vi "main.vi"() -> ()   [LabVIEW 2023, in "Lavatory_Management.lvlib"]
doc: "Airplane lavatory simulator"
uses:
  Lavatory_Management.lvlib
  Controls/Queue Opertaions.ctl
  Controls/Managemet_data.ctl
  Controls/Lavatory_data.ctl
  Queue_Driver.lvlib
panel:
  out "Alarm Time D":dbl caption="Secs" format="%#.3g"
  out "Alarm Time C":dbl caption="Secs" format="%#.3g"
  out "Alarm Time B":dbl caption="Secs" format="%#.3g"
  out "Alarm Time A":dbl caption="Secs" format="%#.3g"
  in  "error in (no error)":errorcluster
  in  "Stop simulation":bool
  in  "Alarm Timer Limit":i32=10 caption="secs" min=1 max=120 step=1
  in  "Lavatory D Occupied":bool
  in  "Lavatory B Occupied":bool
  in  "Lavatory C Occupied":bool
  in  "Lavatory A Occupied":bool
  in  "Alarm Acknowledge":bool
  out "Lavatory":string
  out "Alarm":bool
  in  "Seatbelt Sign ON":bool
  out "Lavatories_Occupied_Rear":bool caption="Lavatories \nOccupied"
  out "Lavatories_Occupied_Front":bool caption="Lavatories \nOccupied"
  out "Return_to_seat_d":bool caption="Return to seat"
  out "Return_to_seat_b":bool caption="Return to seat"
  out "Return_to_seat_c":bool caption="Return to seat"
  out "Return_to_seat_a":bool caption="Return to seat"
  out "Occupied_C":bool caption="Occupied C"
  out "Occupied_D":bool caption="Occupied D"
  out "Occupied_B":bool caption="Occupied B"
  out "Occupied_A":bool caption="Occupied A"
  # "Airplane Lavatory Signs"
  # "Front"
  # "Rear"
  # "Lavatory A"
  # "Lavatory C"
  # "Lavatory B"
  # "Lavatory D"
  # "Simulation Controls & Indicators"
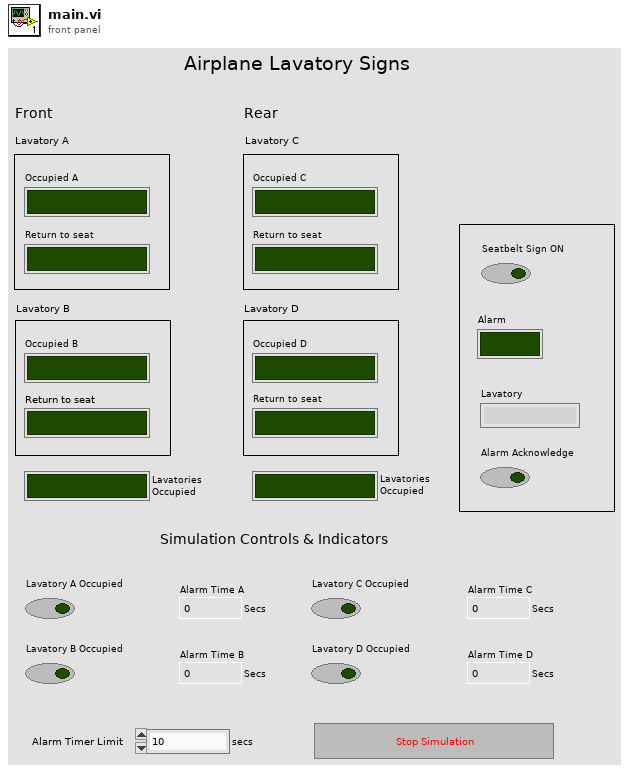
[diagram p1: front panel]
types:
  T1 = typedef "Lavatory_Management.lvlib/Managemet_data.ctl" = cluster{"Lavatory_A":T2, "Lavatory_B":T2, "Lavatory_C":T2, "Lavatory_D":T2, "Seat_belt":bool, "Alarm":bool, "Lavatory":string, "Timr_Limit":i32, "Time_Now":timestamp}
  T2 = typedef "Lavatory_Management.lvlib/Lavatory_data.ctl" = cluster{"Timer":timestamp, "Occupied":bool}
  T3 = typedef "Queue_Driver.lvlib/Queue Opertaions.ctl" = enum16{"Create", "Enqueue", "Enqueue N", "Flush", "Dequeue", "Destroy"}
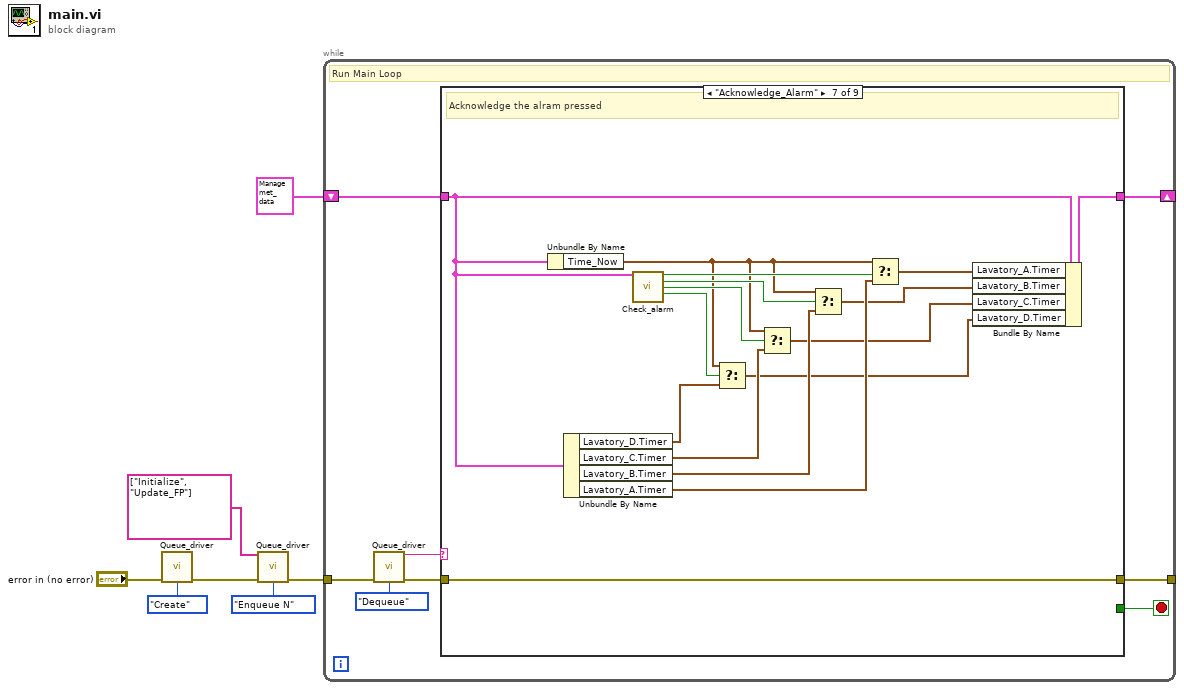
[diagram p0: block diagram]
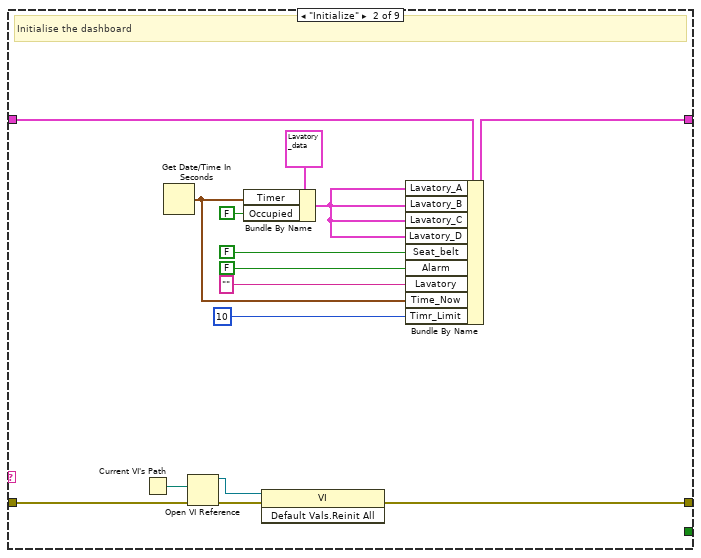
[diagram p3: hidden frame]
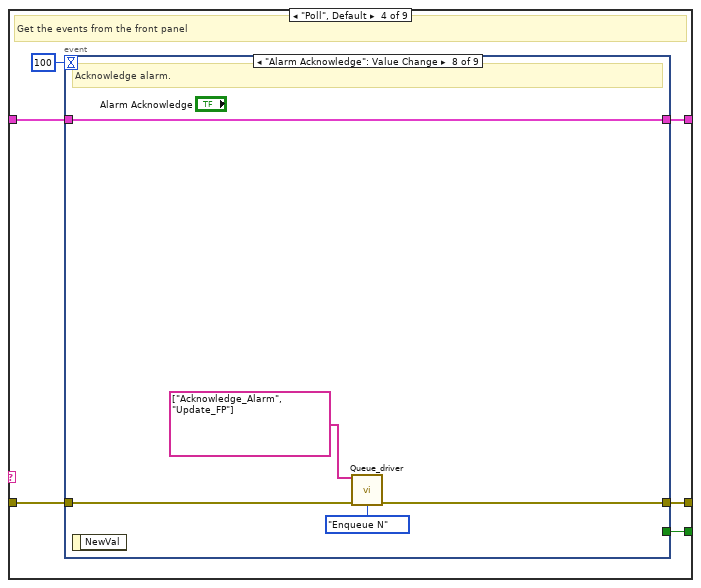
[diagram p5: hidden frame]
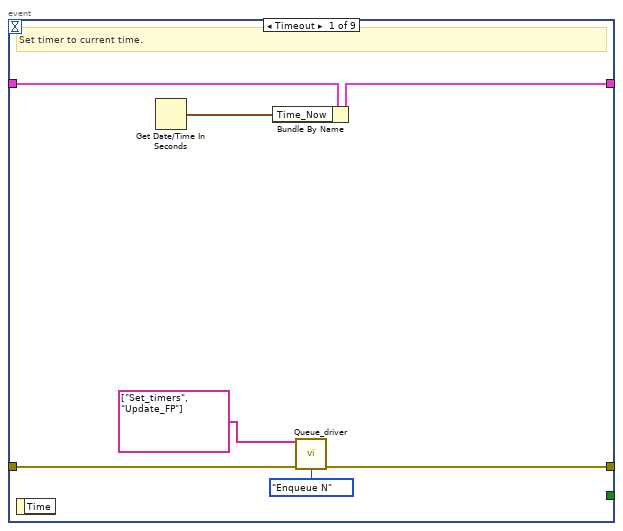
[diagram p6: hidden frame]
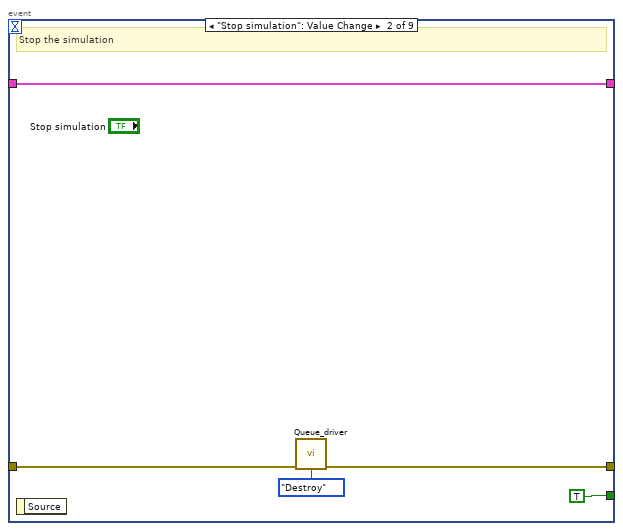
[diagram p7: hidden frame]
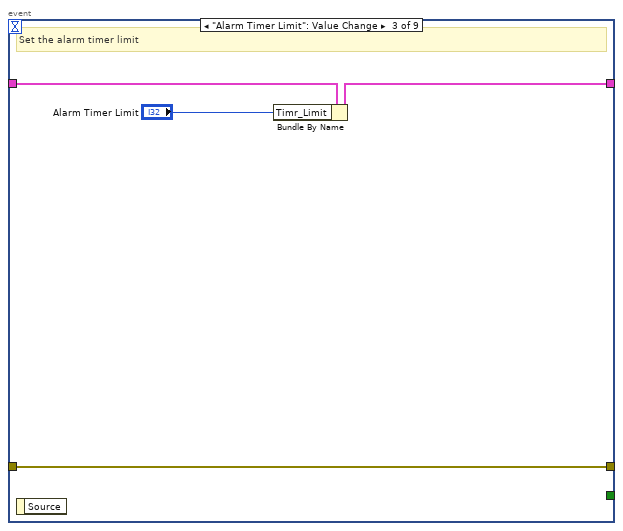
[diagram p8: hidden frame]
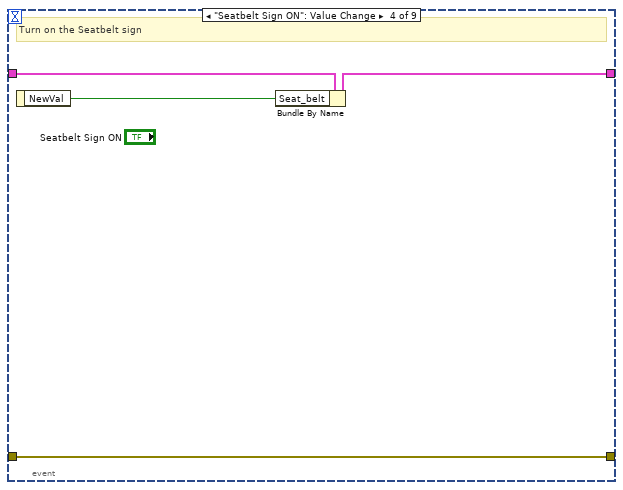
[diagram p9: hidden frame]
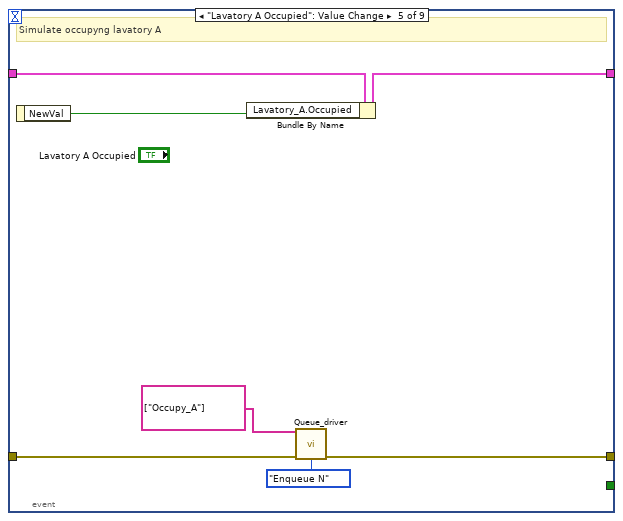
[diagram p10: hidden frame]
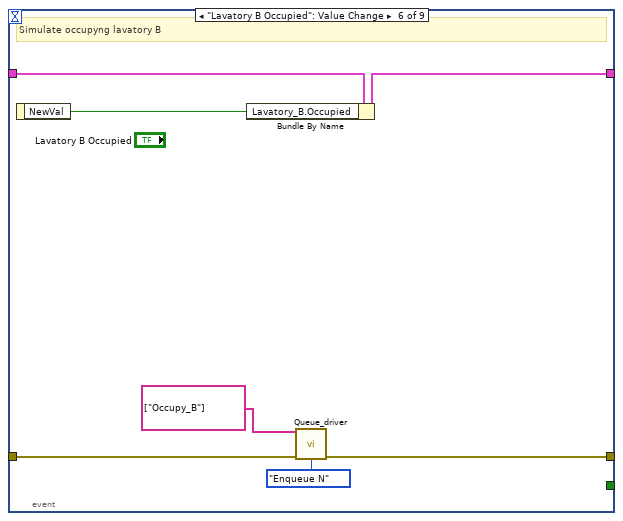
[diagram p11: hidden frame]
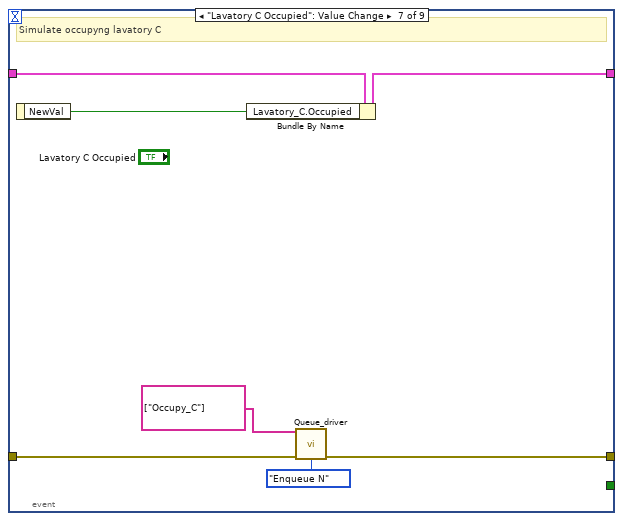
[diagram p12: hidden frame]
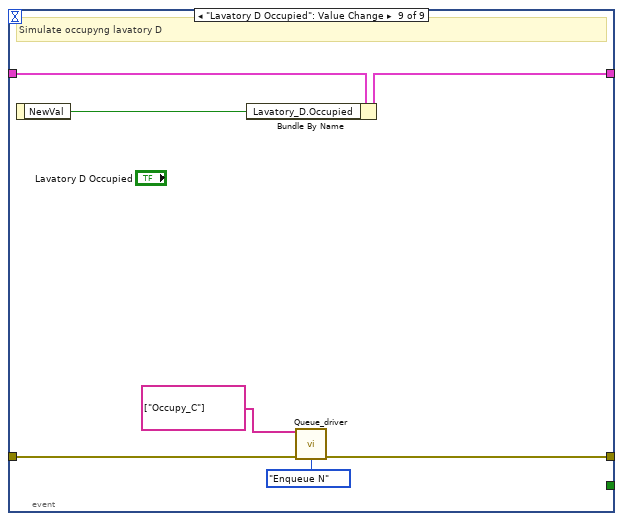
[diagram p13: hidden frame]
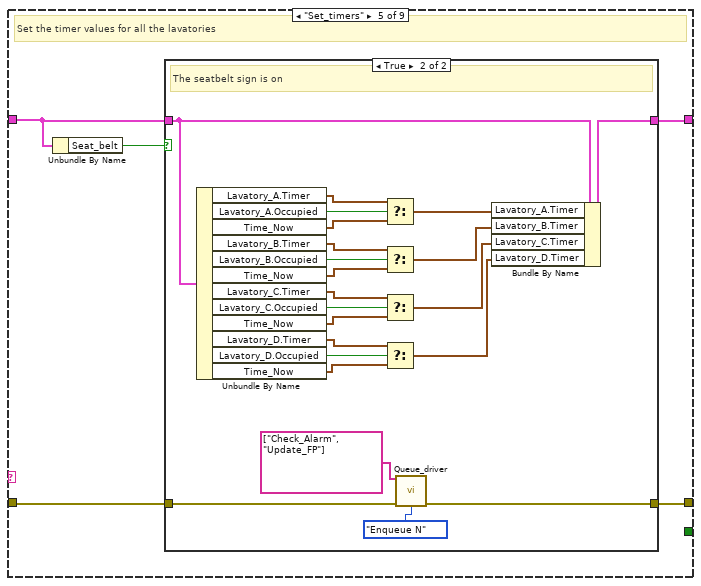
[diagram p14: hidden frame]
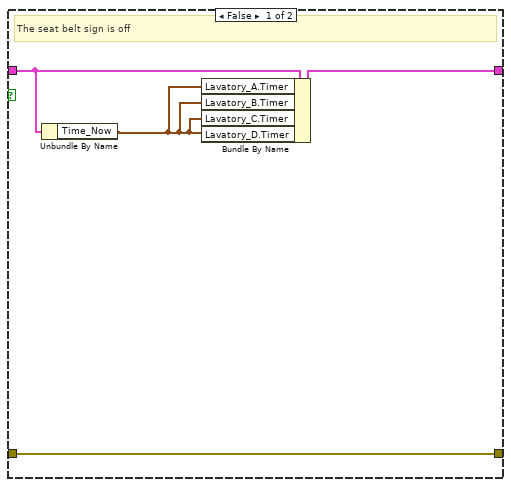
[diagram p15: hidden frame]
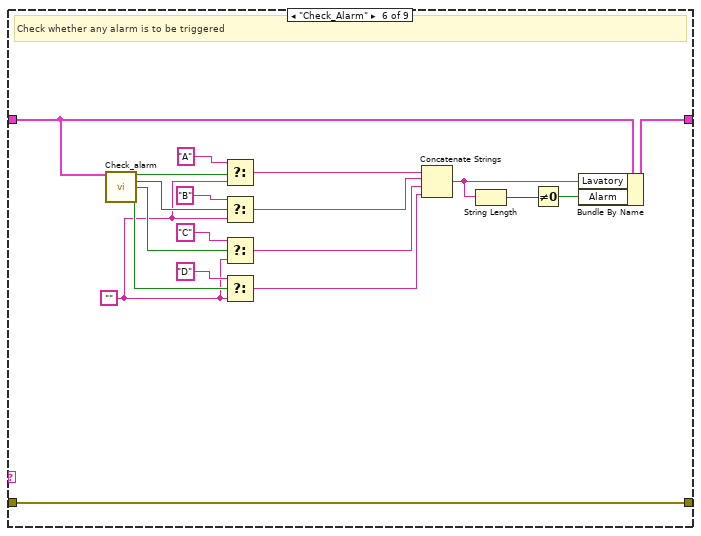
[diagram p16: hidden frame]
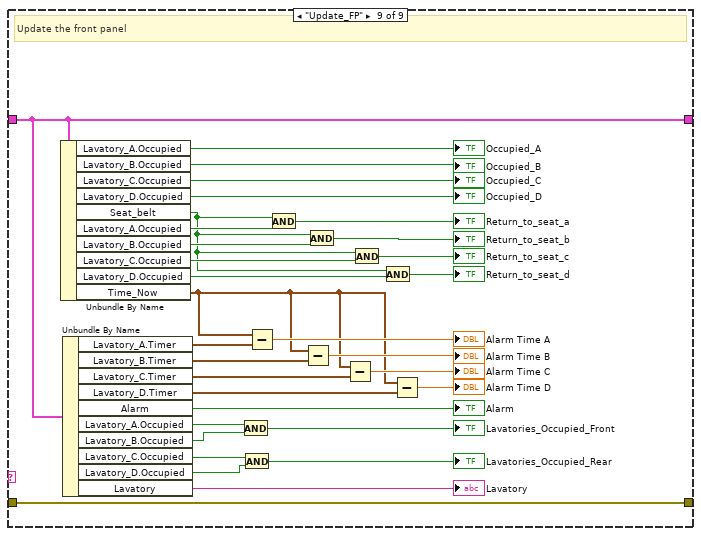
[diagram p18: hidden frame]
diagram:
  n1 = call "Queue_driver.vi"("error in (no error)"="error in (no error)", "Operations"=Queue_Opertaions."Create") -> ("error out"=w5:errorcluster)  [unwired: 12 in, 1 out]
  n2 = call "Queue_driver.vi"("Array Elements"=string[] ["Initialize", "Update_FP"], "error in (no error)"=w5, "Operations"=Queue_Opertaions."Enqueue N") -> ("error out"=w4:errorcluster)  [unwired: 11 in, 1 out]
  n3 = while {
    tunnel: w4 -> [w15]
    tunnel: [w12] -> _
    shift-right: [w9] -> _
    shift-left: T1 {"Lavatory_A"={"Timer"=timestamp(0 s since 1904-01-01), "Occupied"=FALSE}, "Lavatory_B"={"Timer"=timestamp(0 s since 1904-01-01), "Occupied"=FALSE}, "Lavatory_C"={"Timer"=timestamp(0 s since 1904-01-01), "Occupied"=FALSE}, "Lavatory_D"={"Timer"=timestamp(0 s since 1904-01-01), "Occupied"=FALSE}, "Seat_belt"=TRUE, "Alarm"=TRUE, "Lavatory"="", "Timr_Limit"=0, "Time_Now"=timestamp(0 s since 1904-01-01)} -> [w10]
    stop <- w8 stop-if-true
    # "Run Main Loop"
    n4 = call "Queue_driver.vi"("error in (no error)"=w15, "Operations"=Queue_Opertaions."Dequeue") -> ("Element out"=w11:string, "error out"=w13:errorcluster)  [unwired: 12 in]
    n5 = case shown="\"Acknowledge_Alarm\"" w11 {
      tunnel: [w16 w22 w33 w40 w95 w143 w144 w160 w165] -> w12
      tunnel: w13 -> [w16 w32 w33 w39 w94 w143 w144 w160 w165]
      tunnel: w10 -> [w17 w31 w34 w38 w96 w142 w158 w161 w178]
      tunnel: [w17 w30 w34 w37 w97 w141 w149 w161 w178] -> w9
      tunnel: [_ _ _ w36 _ _ _ _ _] -> w8
      frame "/***init***/" {
        # "Contains initialising states"
      }
      frame "Initialize" {
        # "Initialise the dashboard"
        n6 = Current VI's Path() -> (path=w23:path)
        n7 = Get Date/Time In Seconds() -> (seconds since 1Jan1904=w19:timestamp)
        n8 = Open VI Reference(vi path=w23, error in (no error)=w32) -> (vi reference=w21:refnum<vi>, error out=w24:errorcluster)  [unwired: 4 in]
        n9 = Bundle By Name(cluster=T2 {"Timer"=timestamp(0 s since 1904-01-01), "Occupied"=FALSE} ("Cluster"), "Timer"=w19, "Occupied"=FALSE) -> (w25:T2)
        n10 = invoke class="VI" method="Default Vals.Reinit All"(reference=w21, error in=w24) -> (error out=w22:errorcluster)  [unwired: 1 in, 2 out]
        n11 = Bundle By Name(cluster=w31, "Lavatory_A"=w25, "Lavatory_B"=w25, "Lavatory_C"=w25, "Lavatory_D"=w25, "Seat_belt"=FALSE, "Alarm"=FALSE, "Lavatory"="", "Time_Now"=w19, "Timr_Limit"=10) -> (w30:T1)
      }
      frame "/***Functionality***/" {
      }
      frame "Poll", Default {
        # "Get the events from the front panel"
        n12 = event shown="[7] \"Alarm Acknowledge\": Value Change" {
          selector: _ -> [_ _ _ _ _ _ _ _ _]
          dyn-events: _ -> [_ _ _ _ _ _ _ _ _]
          timeout: 100 -> [_ _ _ _ _ _ _ _ _]
          tunnel: [w45 w49 w53 w59 w63 w70 w77 w84 w89] -> w40
          tunnel: w39 -> [w47 w51 w53 w59 w67 w74 w81 w85 w93]
          tunnel: w38 -> [w46 w50 w56 w60 w66 w73 w80 w86 w92]
          tunnel: [w42 w50 w55 w58 w65 w72 w79 w86 w91] -> w37
          tunnel: [_ TRUE _ _ _ _ _ _ _] -> w36
          event Timeout {
            # "Set timer to current time."
            n13 = event-data() -> ()  [unwired: 1 in, 1 out]
            n14 = Get Date/Time In Seconds() -> (seconds since 1Jan1904=w41:timestamp)
            n15 = Bundle By Name(cluster=w46, "Time_Now"=w41) -> (w42:T1)
            n16 = call "Queue_driver.vi"("Array Elements"=string[] ["Set_timers", "Update_FP"], "error in (no error)"=w47, "Operations"=Queue_Opertaions."Enqueue N") -> ("error out"=w45:errorcluster)  [unwired: 11 in, 1 out]
          }
          event "Stop simulation": Value Change {
            # "Stop the simulation"
            n17 = event-data() -> ()  [unwired: 1 in, 1 out]
            n18 = call "Queue_driver.vi"("error in (no error)"=w51, "Operations"=Queue_Opertaions."Destroy") -> ("error out"=w49:errorcluster)  [unwired: 12 in, 1 out]
          }
          event "Alarm Timer Limit": Value Change {
            # "Set the alarm timer limit"
            n19 = event-data() -> ()  [unwired: 1 in, 1 out]
            n20 = Bundle By Name(cluster=w56, "Timr_Limit"="Alarm Timer Limit") -> (w55:T1)
          }
          event "Seatbelt Sign ON": Value Change {
            # "Turn on the Seatbelt sign"
            n21 = event-data() -> ("NewVal"=w57:bool)  [unwired: 1 in]
            n22 = Bundle By Name(cluster=w60, "Seat_belt"=w57) -> (w58:T1)
          }
          event "Lavatory A Occupied": Value Change {
            # "Simulate occupyng lavatory A"
            n23 = event-data() -> ("NewVal"=w64:bool)  [unwired: 1 in]
            n24 = Bundle By Name(cluster=w66, "Lavatory_A.Occupied"=w64) -> (w65:T1)
            n25 = call "Queue_driver.vi"("Array Elements"=string[] ["Occupy_A"], "error in (no error)"=w67, "Operations"=Queue_Opertaions."Enqueue N") -> ("error out"=w63:errorcluster)  [unwired: 11 in, 1 out]
          }
          event "Lavatory B Occupied": Value Change {
            # "Simulate occupyng lavatory B"
            n26 = event-data() -> ("NewVal"=w71:bool)  [unwired: 1 in]
            n27 = Bundle By Name(cluster=w73, "Lavatory_B.Occupied"=w71) -> (w72:T1)
            n28 = call "Queue_driver.vi"("Array Elements"=string[] ["Occupy_B"], "error in (no error)"=w74, "Operations"=Queue_Opertaions."Enqueue N") -> ("error out"=w70:errorcluster)  [unwired: 11 in, 1 out]
          }
          event "Lavatory C Occupied": Value Change {
            # "Simulate occupyng lavatory C"
            n29 = event-data() -> ("NewVal"=w78:bool)  [unwired: 1 in]
            n30 = Bundle By Name(cluster=w80, "Lavatory_C.Occupied"=w78) -> (w79:T1)
            n31 = call "Queue_driver.vi"("Array Elements"=string[] ["Occupy_C"], "error in (no error)"=w81, "Operations"=Queue_Opertaions."Enqueue N") -> ("error out"=w77:errorcluster)  [unwired: 11 in, 1 out]
          }
          event "Alarm Acknowledge": Value Change {
            # "Acknowledge alarm."
            n32 = event-data() -> ()  [unwired: 1 in, 1 out]
            n33 = call "Queue_driver.vi"("Array Elements"=string[] ["Acknowledge_Alarm", "Update_FP"], "error in (no error)"=w85, "Operations"=Queue_Opertaions."Enqueue N") -> ("error out"=w84:errorcluster)  [unwired: 11 in, 1 out]
          }
          event "Lavatory D Occupied": Value Change {
            # "Simulate occupyng lavatory D"
            n34 = event-data() -> ("NewVal"=w90:bool)  [unwired: 1 in]
            n35 = Bundle By Name(cluster=w92, "Lavatory_D.Occupied"=w90) -> (w91:T1)
            n36 = call "Queue_driver.vi"("Array Elements"=string[] ["Occupy_C"], "error in (no error)"=w93, "Operations"=Queue_Opertaions."Enqueue N") -> ("error out"=w89:errorcluster)  [unwired: 11 in, 1 out]
          }
        }
      }
      frame "Set_timers" {
        # "Set the timer values for all the lavatories"
        n37 = Unbundle By Name(w96) -> ("Seat_belt"=w98:bool)
        n38 = case shown="True" w98 {
          tunnel: [w102 w121] -> w97
          tunnel: w96 -> [w100 w124]
          tunnel: [w101 w118] -> w95
          tunnel: w94 -> [w101 w119]
          frame False {
            # "The seat belt sign is off"
            n39 = Unbundle By Name(w100) -> ("Time_Now"=w99:timestamp)
            n40 = Bundle By Name(cluster=w100, "Lavatory_A.Timer"=w99, "Lavatory_B.Timer"=w99, "Lavatory_C.Timer"=w99, "Lavatory_D.Timer"=w99) -> (w102:T1)
          }
          frame True {
            # "The seatbelt sign is on"
            n41 = Unbundle By Name(w124) -> ("Lavatory_A.Timer"=w122:timestamp, "Lavatory_A.Occupied"=w123:bool, "Time_Now"=w116:timestamp, "Lavatory_B.Timer"=w115:timestamp, "Lavatory_B.Occupied"=w114:bool, "Time_Now"=w113:timestamp, "Lavatory_C.Timer"=w112:timestamp, "Lavatory_C.Occupied"=w111:bool, "Time_Now"=w110:timestamp, "Lavatory_D.Timer"=w109:timestamp, "Lavatory_D.Occupied"=w108:bool, "Time_Now"=w107:timestamp)
            n42 = Select(t=w122, s=w123, f=w116) -> (s? t:f=w120:timestamp)
            n43 = Select(t=w115, s=w114, f=w113) -> (s? t:f=w106:timestamp)
            n44 = Select(t=w112, s=w111, f=w110) -> (s? t:f=w105:timestamp)
            n45 = Select(t=w109, s=w108, f=w107) -> (s? t:f=w104:timestamp)
            n46 = call "Queue_driver.vi"("Array Elements"=string[] ["Check_Alarm", "Update_FP"], "error in (no error)"=w119, "Operations"=Queue_Opertaions."Enqueue N") -> ("error out"=w118:errorcluster)  [unwired: 11 in, 1 out]
            n47 = Bundle By Name(cluster=w124, "Lavatory_A.Timer"=w120, "Lavatory_B.Timer"=w106, "Lavatory_C.Timer"=w105, "Lavatory_D.Timer"=w104) -> (w121:T1)
          }
        }
      }
      frame "Check_Alarm" {
        w129 = ""
        # "Check whether any alarm is to be triggered"
        n48 = call "Check_alarm.vi"("Data_Control"=w142) -> ("Trigger A"=w133:bool, "Trigger B"=w131:bool, "Trigger C"=w132:bool, "Trigger D"=w130:bool)  [unwired: 11 in]
        n49 = Select(t="A", s=w133, f=w129) -> (s? t:f=w128:string)
        n50 = Select(t="B", s=w131, f=w129) -> (s? t:f=w127:string)
        n51 = Select(t="C", s=w132, f=w129) -> (s? t:f=w126:string)
        n52 = Select(t="D", s=w130, f=w129) -> (s? t:f=w125:string)
        n53 = Concatenate Strings(w128, w127, w126, w125) -> (w140:string)
        n54 = String Length(string=w140) -> (length=w138:i32)
        n55 = Not Equal To 0?(x=w138) -> (x != 0?=w139:bool)
        n56 = Bundle By Name(cluster=w142, "Lavatory"=w140, "Alarm"=w139) -> (w141:T1)
      }
      frame "Acknowledge_Alarm" {
        # "Acknowledge the alram pressed"
        n57 = Unbundle By Name(w158) -> ("Time_Now"=w153:timestamp)
        n58 = Unbundle By Name(w158) -> ("Lavatory_D.Timer"=w150:timestamp, "Lavatory_C.Timer"=w151:timestamp, "Lavatory_B.Timer"=w152:timestamp, "Lavatory_A.Timer"=w157:timestamp)
        n59 = call "Check_alarm.vi"("Data_Control"=w158) -> ("Trigger A"=w159:bool, "Trigger B"=w156:bool, "Trigger C"=w155:bool, "Trigger D"=w154:bool)  [unwired: 11 in]
        n60 = Select(t=w153, s=w154, f=w150) -> (s? t:f=w145:timestamp)
        n61 = Select(t=w153, s=w155, f=w151) -> (s? t:f=w146:timestamp)
        n62 = Select(t=w153, s=w156, f=w152) -> (s? t:f=w147:timestamp)
        n63 = Select(t=w153, s=w159, f=w157) -> (s? t:f=w148:timestamp)
        n64 = Bundle By Name(cluster=w158, "Lavatory_A.Timer"=w148, "Lavatory_B.Timer"=w147, "Lavatory_C.Timer"=w146, "Lavatory_D.Timer"=w145) -> (w149:T1)
      }
      frame "/***Update front panels***/" {
        # "Update the fornt panel data"
      }
      frame "Update_FP" {
        # "Update the front panel"
        n65 = Unbundle By Name(w178) -> ("Lavatory_A.Occupied"=→"Occupied_A":bool, "Lavatory_B.Occupied"=→"Occupied_B":bool, "Lavatory_C.Occupied"=→"Occupied_C":bool, "Lavatory_D.Occupied"=→"Occupied_D":bool, "Seat_belt"=w185:bool, "Lavatory_A.Occupied"=w189:bool, "Lavatory_B.Occupied"=w188:bool, "Lavatory_C.Occupied"=w187:bool, "Lavatory_D.Occupied"=w186:bool, "Time_Now"=w162:timestamp)
        n66 = Unbundle By Name(w178) -> ("Lavatory_A.Timer"=w171:timestamp, "Lavatory_B.Timer"=w170:timestamp, "Lavatory_C.Timer"=w169:timestamp, "Lavatory_D.Timer"=w168:timestamp, "Alarm"=→"Alarm":bool, "Lavatory_A.Occupied"=w176:bool, "Lavatory_B.Occupied"=w175:bool, "Lavatory_C.Occupied"=w174:bool, "Lavatory_D.Occupied"=w173:bool, "Lavatory"=→"Lavatory":string)
        n67 = And(x=w176, y=w175) -> (x .and. y?=→"Lavatories_Occupied_Front":bool)
        n68 = And(x=w174, y=w173) -> (x .and. y?=→"Lavatories_Occupied_Rear":bool)
        n69 = Subtract(x=w162, y=w171) -> (x-y=→"Alarm Time A":dbl)
        n70 = And(x=w185, y=w189) -> (x .and. y?=→"Return_to_seat_a":bool)
        n71 = Subtract(x=w162, y=w170) -> (x-y=→"Alarm Time B":dbl)
        n72 = And(x=w185, y=w188) -> (x .and. y?=→"Return_to_seat_b":bool)
        n73 = Subtract(x=w162, y=w169) -> (x-y=→"Alarm Time C":dbl)
        n74 = And(x=w185, y=w187) -> (x .and. y?=→"Return_to_seat_c":bool)
        n75 = And(x=w185, y=w186) -> (x .and. y?=→"Return_to_seat_d":bool)
        n76 = Subtract(x=w162, y=w168) -> (x-y=→"Alarm Time D":dbl)
      }
    }
  }
